vi "Ball Intake SS Safety.vi"(11 "Ball Intake Actuator In":T1) -> (3 "Ball Intake Actuator Out":T1)   [LabVIEW 2016]
uses:
  Ball Intake Actuator Out.ctl
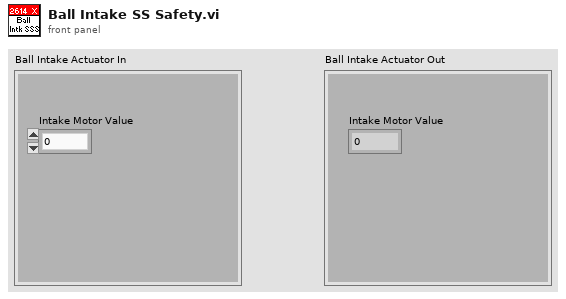
[diagram p1: front panel]
types:
  T1 = typedef "Ball Intake Actuator Out.ctl" = cluster{"Intake Motor Value":dbl}
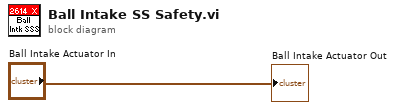
[diagram p0: block diagram]
diagram:
  "Ball Intake Actuator Out" <- "Ball Intake Actuator In"
